vi "To JSON.vi"(6 "Pretty Print?":bool, 8 "error in (no error)":errorcluster, 11 "Type in":refnum<class "Abs_Boolean_1D.lvclass">) -> (0 "error out":errorcluster, 2 "JSON":string, 3 "Type out":refnum<class "Abs_Boolean_1D.lvclass">)   [LabVIEW 2021, in "Abs_Boolean_1D.lvclass"]
uses:
  Abs_Boolean_1D.lvclass
  C:/Program Files (x86)/National Instruments/LabVIEW 2021/vi.lib/TSA/Abstract Data Classes/Abs_Types/Type/Abs_Type.lvclass
  8215d62a-1772-4c04-9c96-c277d69791cc.vi
  <vilib>/Utility/LVClass/Get LV Class Name.vi
  <vilib>/JDP Science/JSONtext/Variant to JSON Text.vi
  <vilib>/JDP Science/JSONtext/Set Multiple Object Items.vi
  Array 1D/Abs_Array1D.lvclass
  <vilib>/JDP Science/JSONtext/LVClass Serializer/JSONtext LVClass Serializer.lvclass
  Type/Abs_Type.lvclass
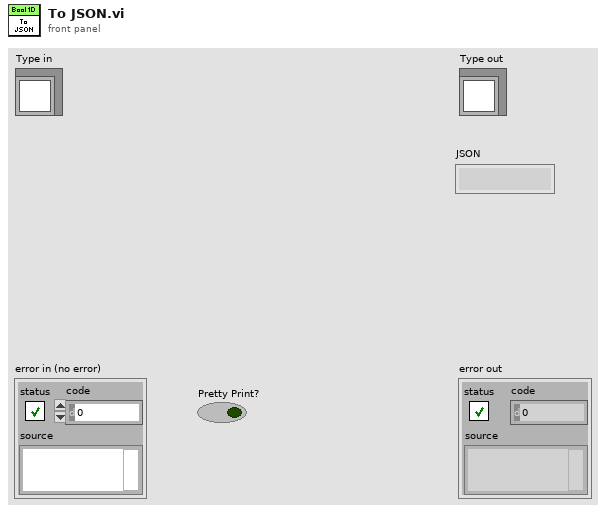
[diagram p1: front panel]
types:
  T1 = typedef "Abs_Boolean_1D.lvclass/Element Type.ctl" = bool
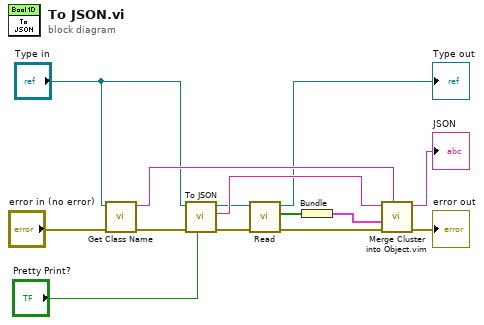
[diagram p0: block diagram]
diagram:
  n1 = call "Get Class Name.vi"("error in (no error)"="error in (no error)", "Abs_Type in"="Type in") -> ("error out"=w10:errorcluster, "class name"=w12:string)  [unwired: 8 in]
  n2 = call-parent "To JSON.vi"("Pretty Print?"="Pretty Print?", "error in (no error)"=w10, "Type in"="Type in") -> ("error out"=w9:errorcluster, "JSON"=w11:string, "Type out"=w7:refnum<class "Abs_Boolean_1D.lvclass">)  [unwired: 6 in]
  n3 = call-dynamic "Read.vi"("error in (no error)"=w9, "Boolean in"=w7) -> ("error out"=w8:errorcluster, "Boolean 1D"=w13:T1[], "Boolean out"=→"Type out":refnum<class "Abs_Boolean_1D.lvclass">)  [unwired: 7 in]
  n4 = Bundle("Boolean 1D"=w13) -> (w14:cluster{"Boolean 1D":T1[]})  [unwired: 1 in]
  n5 = call "Merge Cluster into Object.vim"("$Path or Item Name"=w12, "error in (no error)"=w8, "Any Cluster"=w14, "JSON"=w11) -> ("error out"=→"error out":errorcluster, "<JSON>"=→"JSON":string)  [unwired: 5 in]
